vi "Configure Current Range.vi"(0 "VISA resource name":refnum<visa-resource-name>, 1 "Range Type (1: Custom)":dbl(ring)=1.0 format="%_1g" items=["ALL", "Custom"], 2 "Enable Auto Range (F: Disable)":bool, 5 "Range Configuration (True)":bool[](array[boolean])=[FALSE, FALSE, FALSE, FALSE, FALSE, FALSE, FALSE, TRUE, TRUE, TRUE, TRUE, TRUE, FALSE], 7 "Enable Peak Over Jump (F: Disable)":bool, 9 "Jump Range (20 <10> A)":dbl(ring)=10.0 items=["5m <2.5m>"=0.0025, "10m <5m>"=0.005, "20m <10m>"=0.01, "50m <25m>"=0.025, "100m <50m>"=0.05, "200m <100m>"=0.1, "500m <250m>"=0.25, "1 <500m>"=0.5, "2 <1>"=1.0, "5 <2.5>"=2.5, "10 <5>"=5.0, "20 <10>"=10.0, "40 <20>"=20.0], 11 "error in (no error)":errorcluster, 12 "Manual Range (20 <10> A)":dbl(ring)=10.0 items=["5m <2.5m>"=0.0025, "10m <5m>"=0.005, "20m <10m>"=0.01, "50m <25m>"=0.025, "100m <50m>"=0.05, "200m <100m>"=0.1, "500m <250m>"=0.25, "1 <500m>"=0.5, "2 <1>"=1.0, "5 <2.5>"=2.5, "10 <5>"=5.0, "20 <10>"=10.0, "40 <20>"=20.0]) -> (4 "VISA resource name out":refnum<visa-resource-name>, 15 "error out":errorcluster)   [LabVIEW 2016, in "Yokogawa WT300 Series.lvlib"]
doc: "Configures the current range features."
uses:
  Yokogawa WT300 Series.lvlib
panel:
  # "5m <2.5m> A"
  # "10m <5m> A"
  # "20m <10m> A"
  # "50m <25m> A"
  # "100m <50m> A"
  # "200m <100m> A"
  # "500m <250m> A"
  # "1 <500m> A"
  # "2 <1> A"
  # "5 <2.5> A"
  # "10 <5> A"
  # "20 <10> A"
  # "40 <20> A"
  # "A"
  # "A"
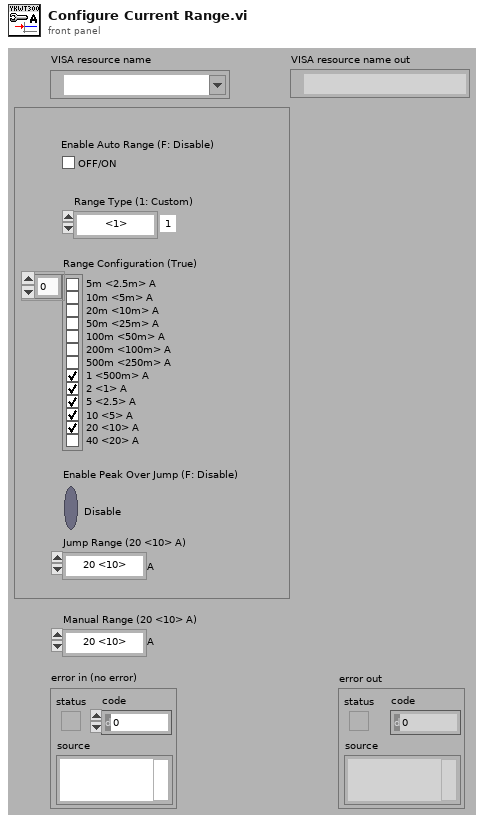
[diagram p1: front panel]
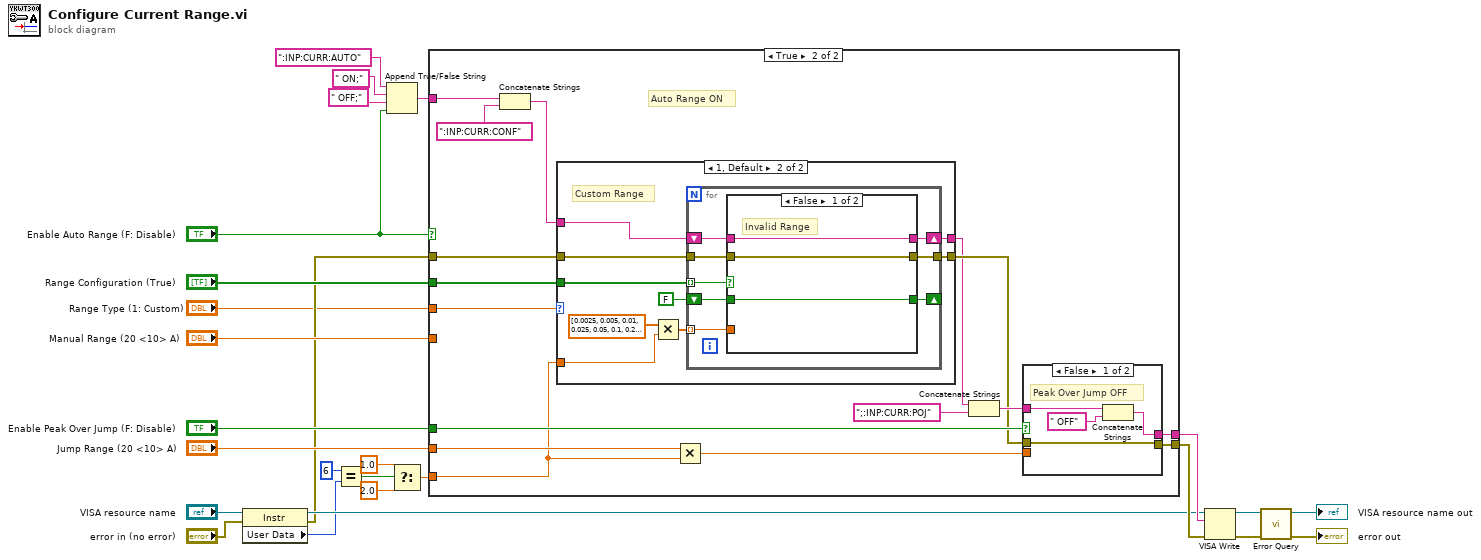
[diagram p0: block diagram]
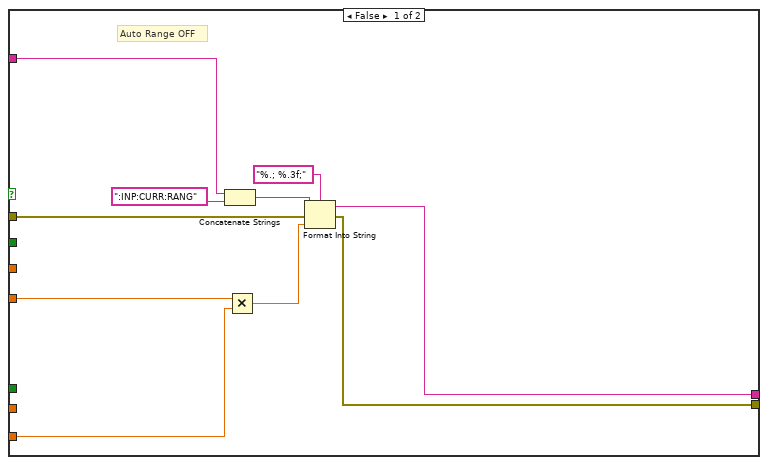
[diagram p2: hidden frame]
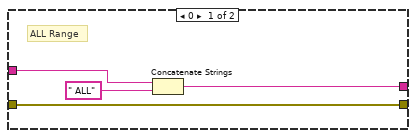
[diagram p3: hidden frame]
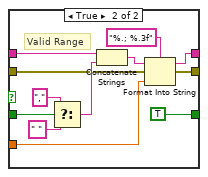
[diagram p4: hidden frame]
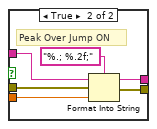
[diagram p5: hidden frame]
diagram:
  n1 = property class="Instr"(reference="VISA resource name", error in="error in (no error)") -> (reference out=w6:refnum<visa-resource-name>, error out=w5:errorcluster, "User Data"=w4:u32)
  n2 = Equal?(x=i64 6 ("y"), y=w4) -> (x = y?=w17:bool)
  n3 = Append True/False String ("True/False 文字列を追加")(1:"Enable Auto Range (F: Disable)", 2:" OFF;", 3:" ON;", 4:":INP:CURR:AUTO") -> (0:w13:string)
  n4 = Select(t=1.0 ("y"), s=w17, f=2.0 ("y")) -> (s? t:f=w15:dbl)
  n5 = case shown="True" "Enable Auto Range (F: Disable)" {
    tunnel: "Manual Range (20 <10> A)" -> [w33 _]
    tunnel: w15 -> [w32 w47]
    tunnel: "Range Configuration (True)" -> [_ w52]
    tunnel: w13 -> [w30 w41]
    tunnel: "Enable Peak Over Jump (F: Disable)" -> [_ w51]
    tunnel: "Jump Range (20 <10> A)" -> [_ w48]
    tunnel: [w29 w39] -> w10
    tunnel: w5 -> [w28 w46]
    tunnel: [w27 w45] -> w9
    tunnel: "Range Type (1: Custom)" -> [_ w42]
    frame False {
      # "Auto Range OFF"
      n6 = Concatenate Strings(w30, ":INP:CURR:RANG") -> (w36:string)
      n7 = Multiply(x=w33, y=w32) -> (x*y=w34:dbl)
      n8 = Format Into String(format string="%.; %.3f;" ("Œ`Ž®•¶Žš—ñ"), initial string=w36, error in=w28, w34) -> (resulting string=w29:string, error out=w27:errorcluster)
    }
    frame True {
      # "Auto Range ON"
      n9 = Concatenate Strings(w41, ":INP:CURR:CONF") -> (w37:string)
      n10 = case shown="1, Default" w42 {
        tunnel: w52 -> [_ w65]
        tunnel: [w54 w62] -> w38
        tunnel: w47 -> [_ w57]
        tunnel: w46 -> [w56 w61]
        tunnel: [w56 w60] -> w44
        tunnel: w37 -> [w53 w58]
        frame 0 {
          # "ALL Range"
          n11 = Concatenate Strings(w53, " ALL") -> (w54:string)
        }
        frame 1, Default {
          # "Custom Range"
          n12 = Multiply(x=dbl[] [0.0025, 0.005, 0.01, 0.025, 0.05, 0.1, 0.25, 0.5, 1.0, 2.5, 5.0, 10.0, 20.0], y=w57) -> (x*y=w63:dbl[])
          n13 = for {
            tunnel: w65 -> [w71] mode=indexing
            shift-right: [w72] -> w62
            shift-left: w58 -> [w73]
            tunnel: w63 -> [w70] mode=indexing
            tunnel: w61 -> [w69]
            tunnel: [w68] -> w60
            shift-right: [w66] -> _
            shift-left: FALSE -> [w67]
            n14 = case shown="False" w71 {
              tunnel: w73 -> [w76 w86]
              tunnel: [w76 w82] -> w72
              tunnel: w70 -> [_ w81]
              tunnel: w69 -> [w75 w80]
              tunnel: [w75 w77] -> w68
              tunnel: w67 -> [w74 w79]
              tunnel: [w74 TRUE] -> w66
              frame False {
                # "Invalid Range"
              }
              frame True {
                # "Valid Range"
                n15 = Select(t=",", s=w79, f=" ") -> (s? t:f=w85:string)
                n16 = Concatenate Strings(w86, w85) -> (w84:string)
                n17 = Format Into String(format string="%.; %.3f" ("Œ`Ž®•¶Žš—ñ"), initial string=w84, error in=w80, w81) -> (resulting string=w82:string, error out=w77:errorcluster)
              }
            }
          }
        }
      }
      n18 = Multiply(x=w48, y=w47) -> (x*y=w49:dbl)
      n19 = Concatenate Strings(w38, ";:INP:CURR:POJ") -> (w50:string)
      n20 = case shown="False" w51 {
        tunnel: w50 -> [w91 w97]
        tunnel: w49 -> [_ w96]
        tunnel: [w90 w95] -> w39
        tunnel: [w89 w94] -> w45
        tunnel: w44 -> [w89 w93]
        frame False {
          # "Peak Over Jump OFF"
          n21 = Concatenate Strings(w91, " OFF" ("•¶Žš—ñ")) -> (w90:string)
        }
        frame True {
          # "Peak Over Jump ON"
          n22 = Format Into String(format string="%.; %.2f;" ("Œ`Ž®•¶Žš—ñ"), initial string=w97, error in=w93, w96) -> (resulting string=w95:string, error out=w94:errorcluster)
        }
      }
    }
  }
  n23 = VISA Write ("VISA書き込み")(VISA resource name=w6, write buffer=w10, error in (no error)=w9) -> (VISA resource name out=w26:refnum<visa-resource-name>, error out=w25:errorcluster)  [unwired: 1 out]
  n24 = call "Error Query.vi"("error in (no error)"=w25, "VISA resource name"=w26) -> ("error out"=→"error out":errorcluster, "VISA resource name out"=→"VISA resource name out":refnum<visa-resource-name>)  [unwired: 6 in, 2 out]
